vi "2. Load the corresponding configuration by providing the prototype.vi"() -> ()   [LabVIEW 2017]
uses:
  78ed0920-6659-4eda-877b-0f5eba050fac.vi
  718255df-b8d2-40a8-8742-692be2ef38df.vi
  99991f6a-3e05-4112-8a38-efb4fd0ba84e.vi
  6d758480-33f7-47ce-8409-8f97b01b9bf3.vi
  10e7d2c9-10c9-43e7-8e22-890ca59f70a9.vi
  <userlib>/_NEVSTOP/Communicable State Machine(CSM)/addons/API-String-Arugments-Support/_Support/Concatenate Strings If not Empty_csm.vi
  INI-Static-Variable-Support/_Support/FlagInstance-CSMINIVariable.vi
  6d758480-33f7-47ce-8409-8f97b01b9bf3.vi/99de0c97-112a-4c86-9094-c187659127e1.vi
  <userlib>/_NEVSTOP/Communicable State Machine(CSM)/Utility/Build Error Cluster.vi
  10e7d2c9-10c9-43e7-8e22-890ca59f70a9.vi/99de0c97-112a-4c86-9094-c187659127e1.vi
  <userlib>/_NEVSTOP/Communicable State Machine(CSM)/_Support/ChangeFlag/ChangeFlag-Read.vi
  <vilib>/Utility/Data Type/Get Type Information.vi
  <userlib>/_NEVSTOP/Communicable State Machine(CSM)/addons/API-String-Arugments-Support/_Support/Data To SingleElementsArray_csm.vi
  <userlib>/_NEVSTOP/Communicable State Machine(CSM)/addons/API-String-Arugments-Support/_Support/Data To API String Arguments.vi
  INI-Static-Variable-Support/_Support/Parse Used Session and Name.vi
  INI-Static-Variable-Support/_Support/INI-FGV(lvlibp).vi
  INI-Static-Variable-Support/_Support/Populate String with INI Variable.vi
  <userlib>/_NEVSTOP/Communicable State Machine(CSM)/addons/API-String-Arugments-Support/_Support/Convert API String Arguments to Data(variant).vi
  <userlib>/_NEVSTOP/Communicable State Machine(CSM)/addons/API-String-Arugments-Support/_Support/SingleElementsArray To Data_csm.vi
  <userlib>/_NEVSTOP/Communicable State Machine(CSM)/_Support/ChangeFlag/ChangeFlagDB.vi
  INI-Static-Variable-Support/_Support/CSM - Read INI String.vi
  INI-Static-Variable-Support/INI-Static-Variable-Support.lvlib
panel:
  out "address2":cluster{"ip":string, "port":i32}={"ip"="10.144.43.43", "port"=8082}
  out "address1":cluster{"ip":string, "port":i32}={"ip"="10.144.42.42", "port"=8081}
  out "non-existing key":cluster{"ip":string, "port":i32}={"ip"="127.0.0.1", "port"=80}
  out "non-existing section":cluster{"ip":string, "port":i32}={"ip"="127.0.0.1", "port"=80}
  out "existing section":cluster{"ip":string, "port":i32}={"ip"="10.144.41.41", "port"=8080}
  # "read cluster from section"
  # "read cluster from key"
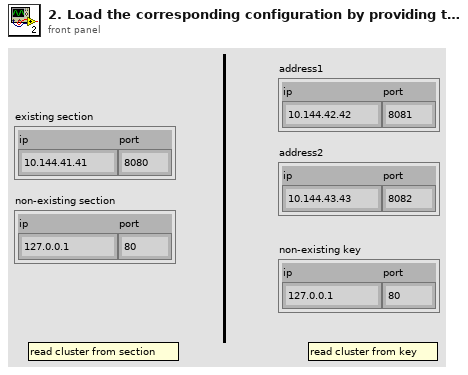
[diagram p1: front panel]
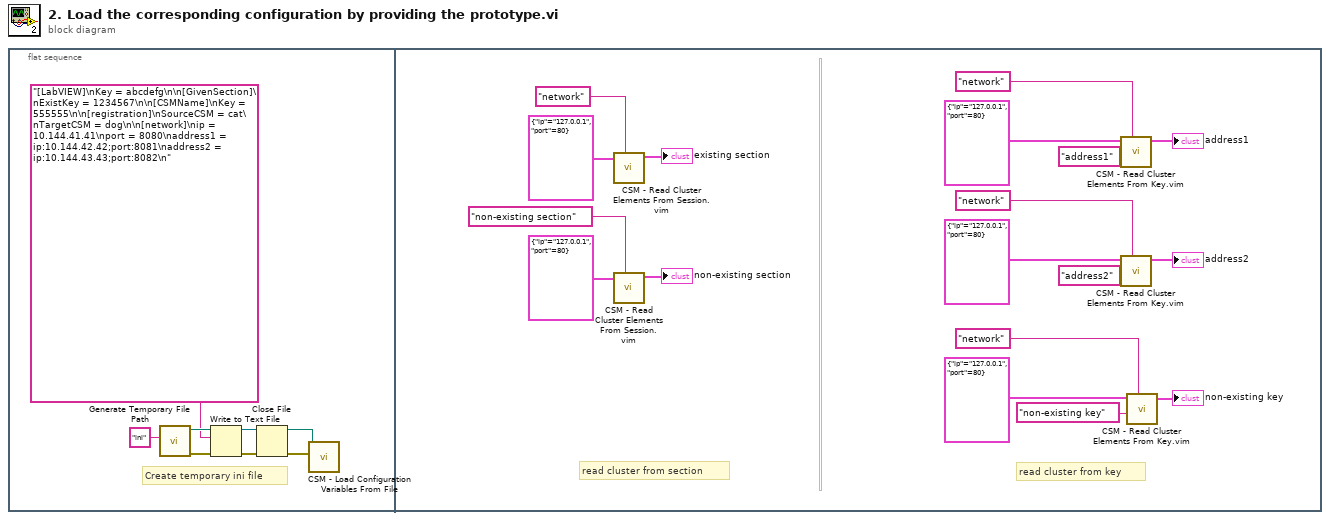
[diagram p0: block diagram]
diagram:
  n1 = flat-sequence {
    frame #0 {
      # "Create temporary ini file"
      n2 = call <vilib>:"Generate Temporary File Path.vi"("Temporary File Extension (tmp)"="ini") -> ("error out"=w8:errorcluster, "Unique Temporary File Path"=w5:path)  [unwired: 9 in]
      n3 = Write to Text File(file (use dialog)=w5, text="[LabVIEW]\nKey = abcdefg\n\n[GivenSection]\nExistKey = 1234567\n\n[CSMName]\nKey = 555555\n\n[registration]\nSourceCSM = cat\nTargetCSM = dog\n\n[network]\nip = 10.144.41.41\nport = 8080\naddress1 = ip:10.144.42.42;port:8081\naddress2 = ip:10.144.43.43;port:8082\n", error in=w8) -> (refnum out=w4:refnum<file>, error out=w6:errorcluster)  [unwired: 1 in, 1 out]
      n4 = Close File(refnum=w4, error in=w6) -> (path=w1:path, error out=w3:errorcluster)
      n5 = call "CSM - Load Configuration Variables From File.vi"("error in (no error)"=w3, "Path"=w1) -> ()  [unwired: 7 in, 1 out]
    }
    frame #1 {
      # "read cluster from section"
      # "read cluster from key"
      n6 = call "CSM - Read Cluster Elements From Session.vim"("Section Name(\"\" as Default)"="network" ("Section Name(\"\" as Default)"), "Cluster"=cluster{"ip":string, "port":i32} {"ip"="127.0.0.1", "port"=80}) -> ("Cluster out"=→"existing section":cluster{"ip":string, "port":i32})  [unwired: 6 in, 1 out]
      n7 = call "CSM - Read Cluster Elements From Session.vim"("Section Name(\"\" as Default)"="non-existing section" ("Section Name(\"\" as Default)"), "Cluster"=cluster{"ip":string, "port":i32} {"ip"="127.0.0.1", "port"=80}) -> ("Cluster out"=→"non-existing section":cluster{"ip":string, "port":i32})  [unwired: 6 in, 1 out]
      n8 = call "CSM - Read Cluster Elements From Key.vim"("Section Name(\"\" as Default)"="network" ("Section Name(\"\" as Default)"), "Key"="address1", "Cluster"=cluster{"ip":string, "port":i32} {"ip"="127.0.0.1", "port"=80}) -> ("Cluster out"=→"address1":cluster{"ip":string, "port":i32})  [unwired: 4 in, 2 out]
      n9 = call "CSM - Read Cluster Elements From Key.vim"("Section Name(\"\" as Default)"="network" ("Section Name(\"\" as Default)"), "Key"="address2", "Cluster"=cluster{"ip":string, "port":i32} {"ip"="127.0.0.1", "port"=80}) -> ("Cluster out"=→"address2":cluster{"ip":string, "port":i32})  [unwired: 4 in, 2 out]
      n10 = call "CSM - Read Cluster Elements From Key.vim"("Section Name(\"\" as Default)"="network" ("Section Name(\"\" as Default)"), "Key"="non-existing key", "Cluster"=cluster{"ip":string, "port":i32} {"ip"="127.0.0.1", "port"=80}) -> ("Cluster out"=→"non-existing key":cluster{"ip":string, "port":i32})  [unwired: 4 in, 2 out]
    }
  }
